vi "test_parse_steps.vi"(8 "error in":errorcluster) -> (0 "error out":errorcluster)   [LabVIEW 2023, in "Easy.SequenceManager.Test.lvlib"]
uses:
  Easy.SequenceManager.Test.lvlib
  src/Step/Step.lvclass
  <vilib>/addons/_JKI Toolkits/Caraya/classes/Assert/Assert Not Error.vi
  <vilib>/addons/_JKI Toolkits/Caraya/classes/Assert/Assert Equal Value and Type_Variant.vi
  <vilib>/addons/_JKI Toolkits/Caraya/classes/Test/Test.lvclass
  <vilib>/addons/_JKI Toolkits/Caraya/classes/Assert/Assert.lvclass
  src/Parameter/Parameter.lvclass
panel:
  # "Connector Pane"
  # "Locals"
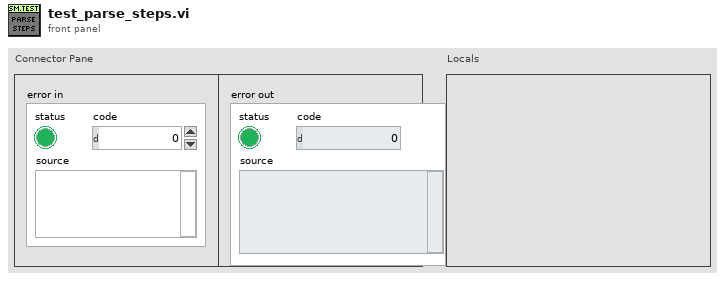
[diagram p1: front panel]
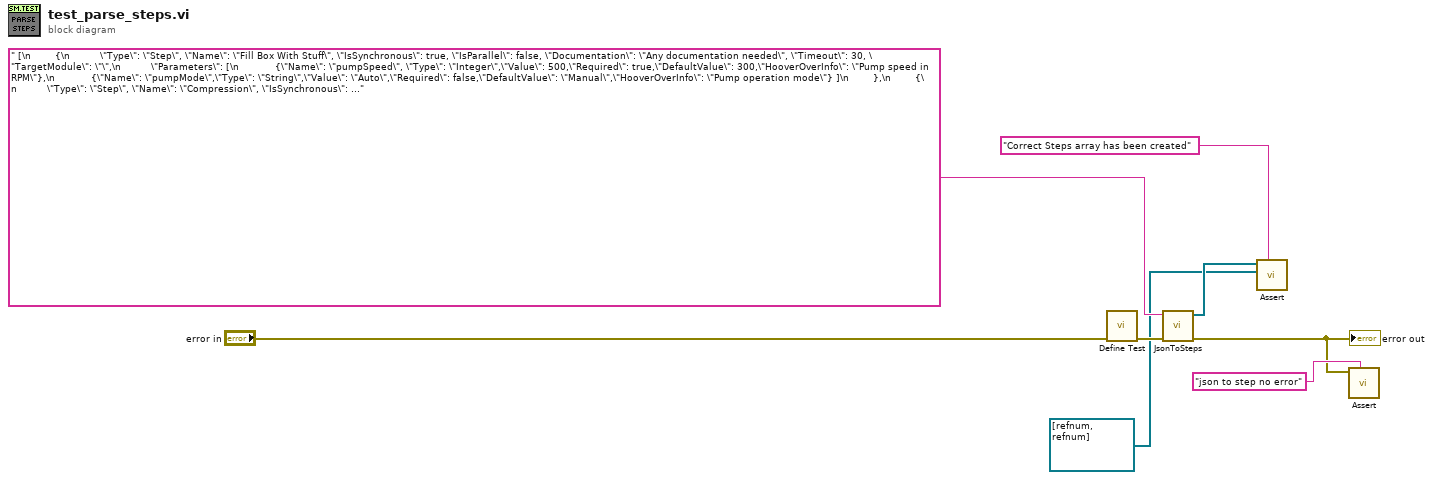
[diagram p0: block diagram]
diagram:
  n1 = call <vilib>:"Define Test.vi"("error in (no error)"="error in") -> ("error out"=w4:errorcluster)  [unwired: 9 in, 1 out]
  n2 = call "JsonToSteps.vi"("error in"=w4, "JSON String"=" [\n        {\n          \"Type\": \"Step\", \"Name\": \"Fill Box With Stuff\", \"IsSynchronous\": true, \"IsParallel\": false, \"Documentation\": \"Any documentation needed\", \"Timeout\": 30, \"TargetModule\": \"\",\n          \"Parameters\": [\n            {\"Name\": \"pumpSpeed\", \"Type\": \"Integer\",\"Value\": 500,\"Required\": true,\"DefaultValue\": 300,\"HooverOverInfo\": \"Pump speed in RPM\"},\n            {\"Name\": \"pumpMode\",\"Type\": \"String\",\"Value\": \"Auto\",\"Required\": false,\"DefaultValue\": \"Manual\",\"HooverOverInfo\": \"Pump operation mode\"} ]\n        },\n        {\n          \"Type\": \"Step\", \"Name\": \"Compression\", \"IsSynchronous\": false, \"IsParallel\": false, \"Documentation\": \"Any documentation needed\", \"Timeout\": 45, \"TargetModule\": \"\",\n          \"Parameters\": [\n            {\"Name\": \"axisTargetPosition1\", \"Type\": \"Float\", \"Value\": 10.5, \"Required\": true, \"DefaultValue\": 0.0, \"HooverOverInfo\": \"Target position for the axis movement\" },\n            {\"Name\": \"axisSpeed1\", \"Type\": \"Float\", \"Value\": 10.5, \"Required\": true, \"DefaultValue\": 0.0, \"HooverOverInfo\": \"Target position for the axis movement\" },\n            {\"Name\": \"axisTargetPosition2\", \"Type\": \"Float\", \"Value\": 10.5, \"Required\": true, \"DefaultValue\": 0.0, \"HooverOverInfo\": \"Target position for the axis movement\"},\n            {\"Name\": \"axisSpeed2\", \"Type\": \"Float\", \"Value\": 10.5, \"Required\": true, \"DefaultValue\": 0.0, \"HooverOverInfo\": \"Target position for the axis movement\"} \n          ]\n        }\n      ]") -> ("error out"=w2:errorcluster, "Steps"=w3:refnum<class "Step.lvclass">[])  [unwired: 7 in, 1 out]
  "error out" <- w2
  n3 = call-poly <vilib>:"Assert.vi"("Label"="Correct Steps array has been created" ("Label (VI Title)"), "Y"=refnum<class "Step.lvclass">[] [refnum, refnum] ("Steps"), "X"=w3) -> ()  [unwired: 7 in, 2 out]
  n4 = call-poly <vilib>:"Assert.vi"("Label"="json to step no error", "Not Error?"=w2) -> ()  [unwired: 8 in, 2 out]
